vi "CLSUIP_Read Replacement class.vi"(1 "VIRetooler.lvclass in":refnum<class "VIRetooler.lvclass">) -> (0 "Replacement class":refnum<vi>)   [LabVIEW 2021, in "MemberVICreation.lvlib" / "VIRetooler.lvclass"]
uses:
  <resource>/Framework/Providers/LVClassLibrary/NewAccessors/VIRetooler/VIRetooler.lvclass
  <resource>/Framework/Providers/LVClassLibrary/NewAccessors/VIRetooler/VIRetooler.lvclass/VIRetooler.ctl
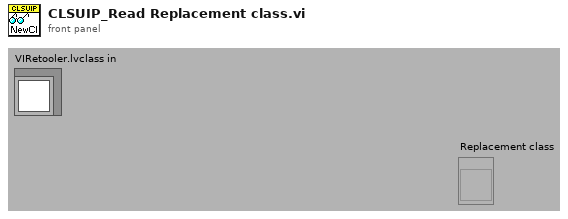
[diagram p1: front panel]
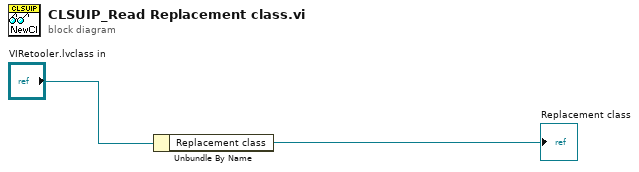
[diagram p0: block diagram]
diagram:
  n1 = Unbundle By Name("VIRetooler.lvclass in") -> ("Replacement class"=→"Replacement class":refnum<vi>)
